vi "temp595.vi"() -> ()   [LabVIEW 2010]
panel:
  out "Waveform Chart":dbl[][](graph)
  in  "stop":bool
  in  "Delay Time (s)":dbl=1.0
  # "Note: Please supply a measured value in volts"
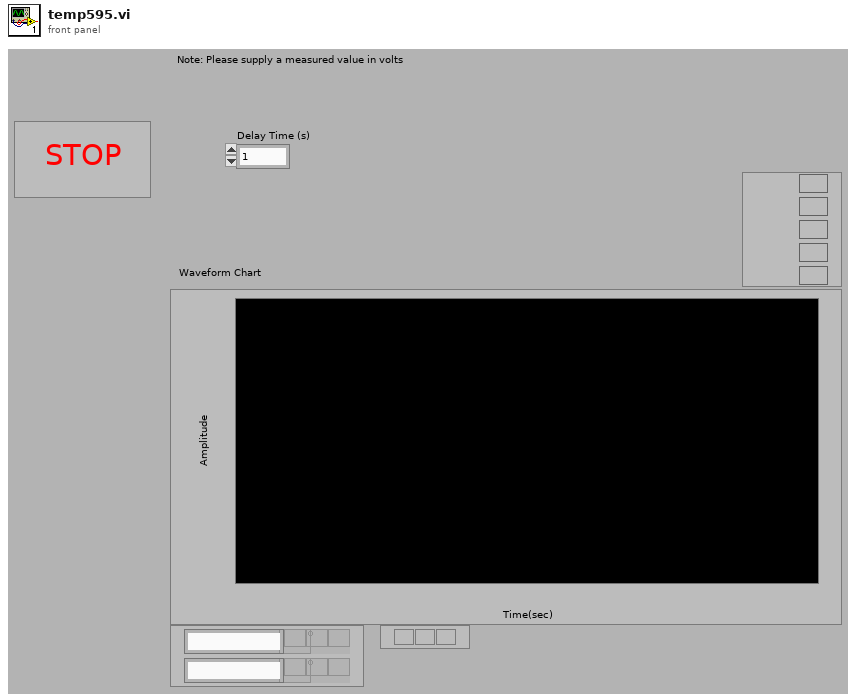
[diagram p1: front panel]
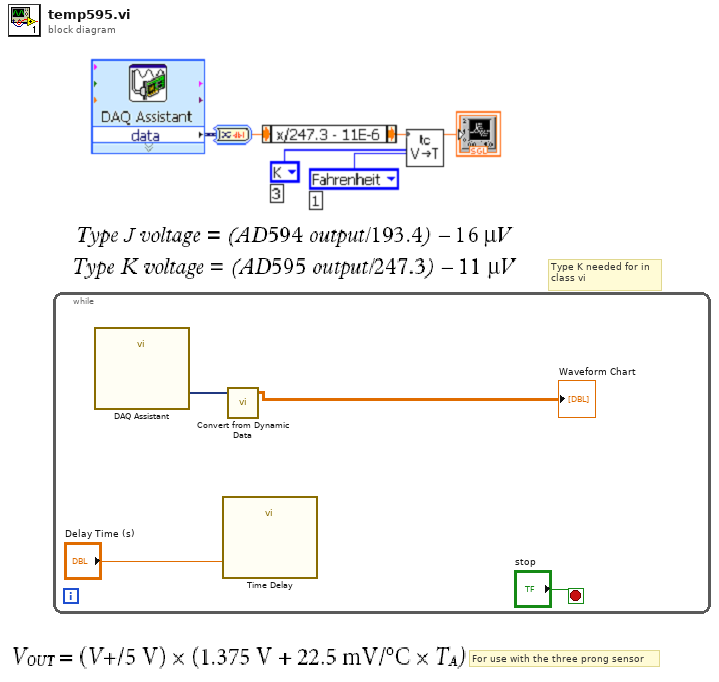
[diagram p0: block diagram]
diagram:
  # "Type K needed for in\nclass vi"
  # "For use with the three prong sensor"
  n1 = while {
    stop <- "stop" stop-if-true
    n2 = call "DAQ Assistant"() -> ("data"=w2:dynamicdata)  [unwired: 17 in, 2 out]
    n3 = call "Time Delay"("Delay Time (s)"="Delay Time (s)") -> ()  [unwired: 10 in, 1 out]
    n4 = call "Convert from Dynamic Data"("Dynamic Data Type"=w2) -> ("Array"=→"Waveform Chart":dbl[][])  [unwired: 3 in]
  }
